vi "brown--constant.vi"() -> (1 "Brown":u32(colorbox))   [LabVIEW 2018]
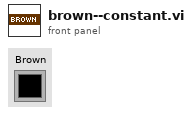
[diagram p1: front panel]
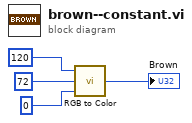
[diagram p0: block diagram]
diagram:
  n1 = call <vilib>:"RGB to Color.vi"("B"=u8 0, "G"=u8 72, "R"=u8 120) -> ("Color"=→"Brown":u32)
